vi "n x n Smooth 2D Array (CSG) v3.vi"(4 "Average":bool caption="Average (F)", 8 "Error In":errorcluster, 9 "Kernel Size":i32=1, 10 "Kernel Type":T1, 11 "Array in":csg[][](array[numeric])) -> (0 "Error Out":errorcluster, 1 "Valid?":bool[][](array[boolean]), 3 "Array out":csg[][](array[numeric]))   [LabVIEW 2021, in "Arrays.lvlib"]
uses:
  Arrays.lvlib
  Kernel Type.ctl
  Time/Time.lvlib
  Utilities/Utilities.lvlib
panel:
  out "elapsed (relative) seconds":dbl
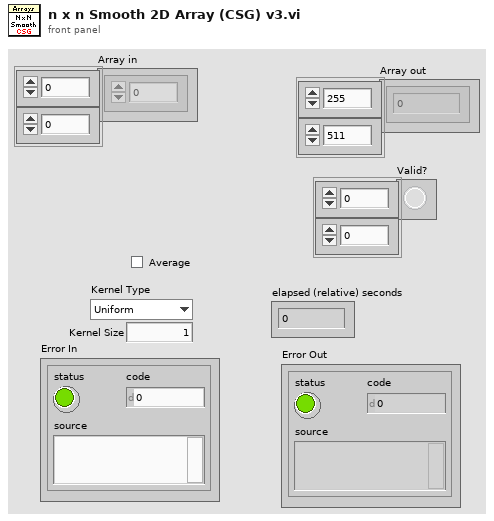
[diagram p1: front panel]
types:
  T1 = typedef "Arrays.lvlib/Kernel Type.ctl" = enum16{"Uniform", "Bilinear", "Gaussian"}
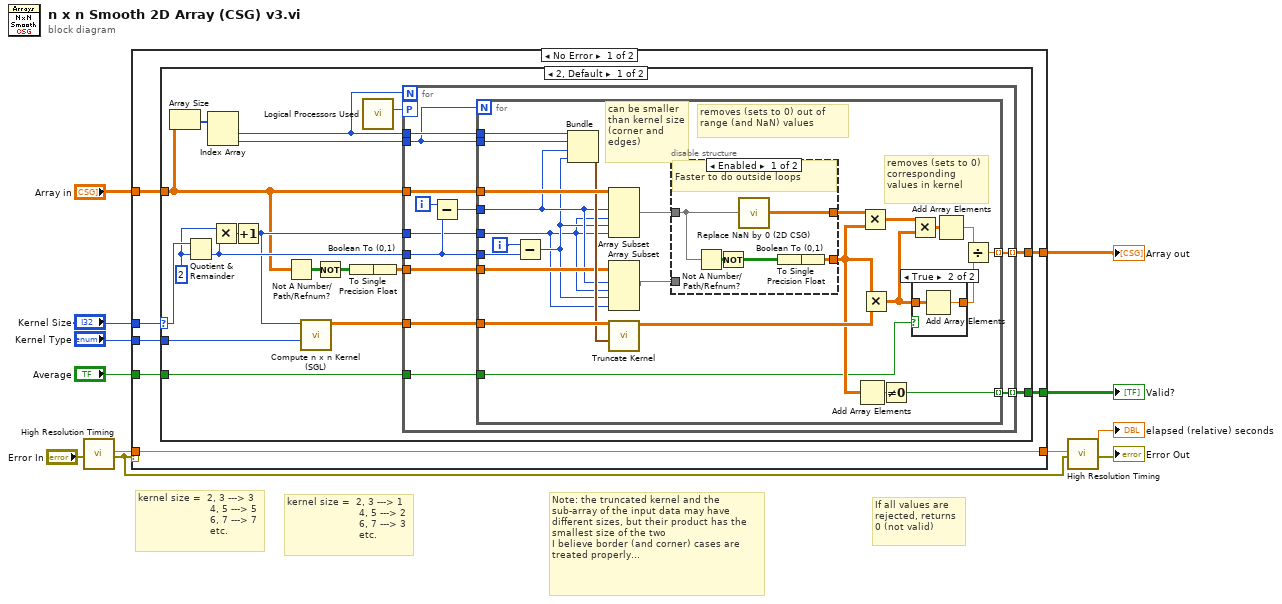
[diagram p0: block diagram]
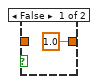
[diagram p2: hidden frame]
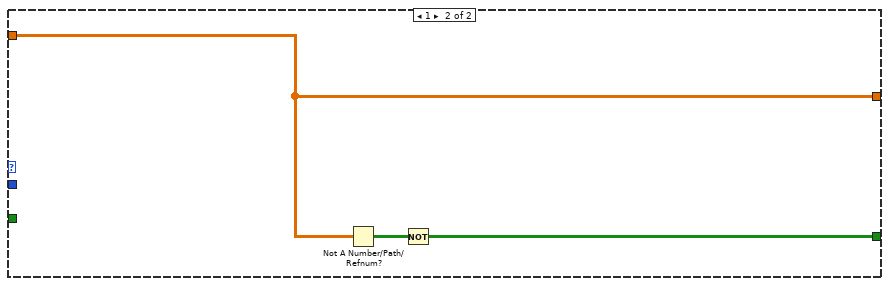
[diagram p4: hidden frame]
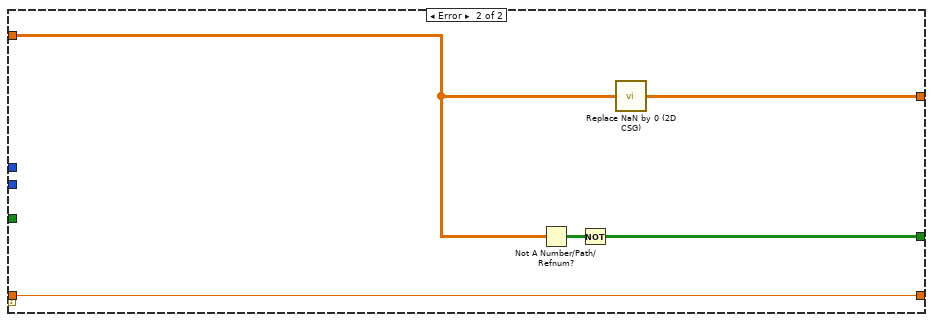
[diagram p5: hidden frame]
diagram:
  # "Note: the truncated kernel and the sub-array of the input data may have different sizes, but their product has the smallest size of the two\nI believe border (and corner) cases are treated properly..."
  # "kernel size =  2, 3 ---> 3\n                        4, 5 ---> 5\n                        6, 7 ---> 7\n                        etc."
  # "kernel size =  2, 3 ---> 1\n                        4, 5 ---> 2\n                        6, 7 ---> 3\n                        etc."
  # "If all values are rejected, returns 0 (not valid)"
  n1 = call "High Resolution Timing.vi"("Error In"="Error In") -> ("elapsed (relative) seconds"=w3:dbl, "Error Out"=w4:errorcluster)  [unwired: 16 in, 1 out]
  n2 = case shown="No Error" w4 {
    tunnel: "Array in" -> [w19 w92]
    tunnel: "Kernel Size" -> [w18 _]
    tunnel: [w17 w93] -> w11
    tunnel: [w16 w91] -> w10
    tunnel: [w13 w90] -> w1
    tunnel: "Kernel Type" -> [w15 _]
    tunnel: "Average" -> [w14 _]
    tunnel: w3 -> [w13 w90]
    frame No Error {
      n3 = case shown="2, Default" w18 {
        selector: w18 -> [w36 _]
        tunnel: w19 -> [w26 w89]
        tunnel: [w33 w89] -> w17
        tunnel: [w29 w87] -> w16
        tunnel: w15 -> [w28 _]
        tunnel: w14 -> [w21 _]
        frame 2, Default {
          w31 = 2 ("y")
          n4 = Array Size(array=w26) -> (size(s)=w38:i32[])
          n5 = Quotient & Remainder(x=w36, y=w31) -> (floor(x/y)=w32:i32)  [unwired: 1 out]
          n6 = Index Array(array=w38) -> (element #1=w35:i32, element #2=w37:i32)  [unwired: 2 in]
          n7 = Multiply(x=w31, y=w32) -> (x*y=w30:i32)
          n8 = Increment(x=w30) -> (x+1=w27:i32)
          n9 = Not A Number/Path/Refnum?(number/path/refnum=w26) -> (NaN/Path/Refnum?=w25:bool[][])
          n10 = call "Compute n x n Kernel (SGL).vi"("Kernel Type"=w28, "Kernel Size"=w27) -> ("Kernel"=w34:sgl[][])  [unwired: 9 in]
          n11 = Not(x=w25) -> (.not. x?=w24:bool[][])
          n12 = Boolean To (0,1)(Boolean=w24) -> (0, 1=w23:i16[][])
          n13 = call "Logical Processors Used.vi"() -> ("# Logical Processor Used"=w20:i32)  [unwired: 6 in]
          n14 = To Single Precision Float(number=w23) -> (single precision float=w22:sgl[][])
          n15 = for {
            N: w35 -> [_]
            tunnel: w26 -> [w50]
            tunnel: w37 -> [w43]
            tunnel: w32 -> [w47]
            tunnel: w27 -> [w46]
            tunnel: w34 -> [w45]
            tunnel: w35 -> [w44]
            tunnel: [w42] -> w33 mode=indexing
            tunnel: [w41] -> w29 mode=indexing
            tunnel: w22 -> [w40]
            tunnel: w21 -> [w39]
            workers-P: w20 -> [_]
            i -> [w49]
            n16 = Subtract(x=w49, y=w47) -> (x-y=w48:i32)
            n17 = for {
              N: w43 -> [_]
              tunnel: w50 -> [w75]
              tunnel: w48 -> [w55]
              tunnel: w47 -> [w73]
              tunnel: w46 -> [w53]
              tunnel: w45 -> [w67]
              tunnel: w44 -> [w72]
              tunnel: w43 -> [w71]
              tunnel: [w68] -> w42 mode=indexing
              tunnel: [w60] -> w41 mode=indexing
              tunnel: w40 -> [w56]
              tunnel: w39 -> [w51]
              i -> [w74]
              # "can be smaller than kernel size (corner and edges)"
              # "removes (sets to 0) corresponding values in kernel"
              # "removes (sets to 0) out of range (and NaN) values"
              n18 = Subtract(x=w74, y=w73) -> (x-y=w54:i32)
              n19 = Bundle(w72, w71, w55, w54) -> (w66:cluster{i32, i32, i32, i32})  [unwired: 1 in]
              n20 = Array Subset(array=w75, index (row)=w55, length (row)=w53, index (col)=w54, length (col)=w53) -> (w59:csg[][])
              n21 = Array Subset(array=w56, index (row)=w55, length (row)=w53, index (col)=w54, length (col)=w53) -> (w52:sgl[][])
              n22 = call "Truncate Kernel.vi"("Array Element Parameters"=w66, "Kernel in"=w67) -> ("Kernel out"=w62:sgl[][])  [unwired: 9 in]
              n23 = disable-structure shown="Enabled" {
                disable-tunnel: w59 -> [w81 w86]
                disable-tunnel: [w82 w85] -> w58
                disable-tunnel: [w80 w86] -> w57
                disable-tunnel: w52 -> [_ w85]
                frame Enabled {
                  # "Faster to do outside loops"
                  n24 = Not A Number/Path/Refnum?(number/path/refnum=w81) -> (NaN/Path/Refnum?=w83:bool[][])
                  n25 = Not(x=w83) -> (.not. x?=w79:bool[][])
                  n26 = call "Replace NaN by 0 (2D CSG).vi"("Array in"=w81) -> ("Array out"=w80:csg[][])  [unwired: 8 in]
                  n27 = Boolean To (0,1)(Boolean=w79) -> (0, 1=w84:i16[][])
                  n28 = To Single Precision Float(number=w84) -> (single precision float=w82:sgl[][])
                }
                frame Disabled {
                }
              }
              n29 = Add Array Elements(numeric array=w58) -> (sum=w63:sgl)
              n30 = Multiply(x=w57, y=w58) -> (x*y=w64:csg[][])
              n31 = Multiply(x=w58, y=w62) -> (x*y=w61:sgl[][])
              n32 = Not Equal To 0?(x=w63) -> (x != 0?=w60:bool)
              n33 = Multiply(x=w64, y=w61) -> (x*y=w65:csg[][])
              n34 = case shown="True" w51 {
                tunnel: [sgl 1.0 w78] -> w69
                tunnel: w61 -> [_ w77]
                frame False {
                }
                frame True {
                  n35 = Add Array Elements(numeric array=w77) -> (sum=w78:sgl)
                }
              }
              n36 = Add Array Elements(numeric array=w65) -> (sum=w70:csg)
              n37 = Divide(x=w70, y=w69) -> (x/y=w68:csg)
            }
          }
        }
        frame 1 {
          n38 = Not A Number/Path/Refnum?(number/path/refnum=w89) -> (NaN/Path/Refnum?=w88:bool[][])
          n39 = Not(x=w88) -> (.not. x?=w87:bool[][])
        }
      }
    }
    frame Error {
      n40 = Not A Number/Path/Refnum?(number/path/refnum=w92) -> (NaN/Path/Refnum?=w94:bool[][])
      n41 = Not(x=w94) -> (.not. x?=w91:bool[][])
      n42 = call "Replace NaN by 0 (2D CSG).vi"("Array in"=w92) -> ("Array out"=w93:csg[][])  [unwired: 8 in]
    }
  }
  "Array out" <- w11
  "Valid?" <- w10
  n43 = call "High Resolution Timing.vi"("relative seconds (NaN)"=w1, "Error In"=w4) -> ("elapsed (relative) seconds"=→"elapsed (relative) seconds":dbl, "Error Out"=→"Error Out":errorcluster)  [unwired: 15 in, 1 out]
